vi "GetBoolFeatureValue.vi"(9 "pFeatureName":string, 10 "handle":i32, 11 "error in (no error)":errorcluster) -> (1 "pBoolValue":i8, 2 "return type":i32, 3 "error out":errorcluster)   [LabVIEW 2016]
uses:
  MVSDKmd.dll
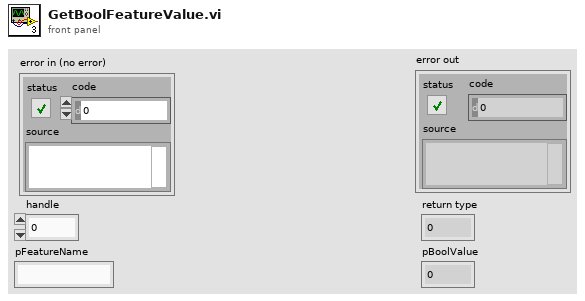
[diagram p1: front panel]
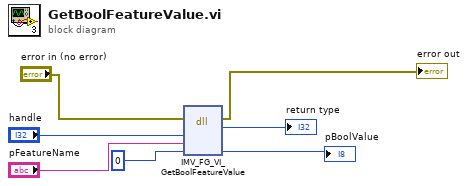
[diagram p0: block diagram]
diagram:
  n1 = dll-call lib="MVSDKmd.dll" fn="IMV_FG_VI_GetBoolFeatureValue"(error in="error in (no error)", "handle"="handle", "pFeatureName"="pFeatureName", "pBoolValue"=i8 0) -> (error out=→"error out":errorcluster, "return type"=→"return type":i32, "pBoolValue"=→"pBoolValue":i8)  [unwired: 4 in, 1 out]
